vi "CTRE_Phoenix_MotorControl_BufferedTrajectoryPointStream_WriteCCI.vi"(8 "error in":errorcluster, 10 "Trajectory Point":T2, 11 "BufferedTrajectoryPointStream_DevRef":T1) -> (0 "error out":errorcluster, 3 "BufferedTrajectoryPointStream_DevRef":T1)   [LabVIEW 2020]
uses:
  <vilib>/Rock Robotics/WPI/ThirdParty/Phoenix-LabVIEW/Motor Controller/Controls/CTRE_Phoenix_MotorControl_MotionProfileTrajectoryPoint.ctl
  <vilib>/Rock Robotics/WPI/ThirdParty/Phoenix-LabVIEW/Motor Controller/Controls/CTRE_Phoenix_MotorControl_BufferedTrajectoryPointStream_DeviceRef.ctl
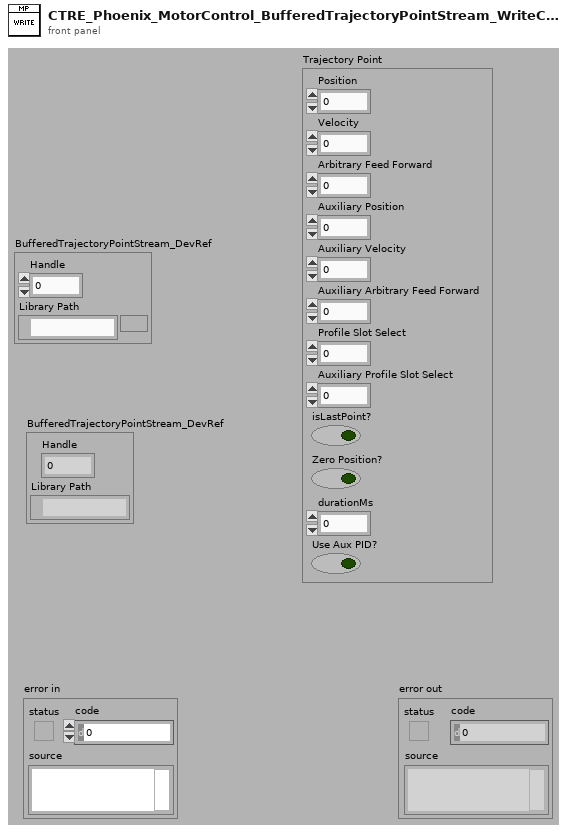
[diagram p1: front panel]
types:
  T1 = typedef "CTRE_Phoenix_MotorControl_BufferedTrajectoryPointStream_DeviceRef.ctl" = cluster{"Handle":u64, "Library Path":path}
  T2 = typedef "CTRE_Phoenix_MotorControl_MotionProfileTrajectoryPoint.ctl" = cluster{"Position":dbl, "Velocity":dbl, "Arbitrary Feed Forward":dbl, "Auxiliary Position":dbl, "Auxiliary Velocity":dbl, "Auxiliary Arbitrary Feed Forward":dbl, "Profile Slot Select":i32, "Auxiliary Profile Slot Select":i32, "isLastPoint?":bool, "Zero Position?":bool, "durationMs":u32, "Use Aux PID?":bool}
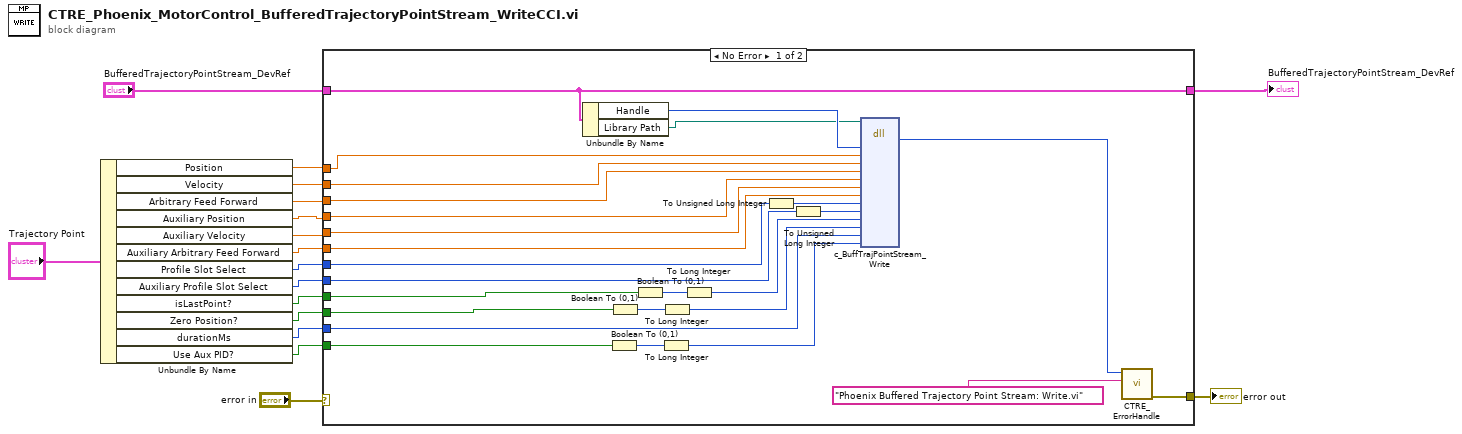
[diagram p0: block diagram]
diagram:
  n1 = Unbundle By Name("Trajectory Point") -> ("Position"=w14:dbl, "Velocity"=w13:dbl, "Arbitrary Feed Forward"=w12:dbl, "Auxiliary Position"=w11:dbl, "Auxiliary Velocity"=w10:dbl, "Auxiliary Arbitrary Feed Forward"=w9:dbl, "Profile Slot Select"=w8:i32, "Auxiliary Profile Slot Select"=w7:i32, "isLastPoint?"=w6:bool, "Zero Position?"=w5:bool, "durationMs"=w4:u32, "Use Aux PID?"=w3:bool)
  n2 = case shown="No Error" "error in" {
    selector: "error in" -> [_ w44]
    tunnel: "BufferedTrajectoryPointStream_DevRef" -> [w20 w45]
    tunnel: [w43 w44] -> w17
    tunnel: [w20 w45] -> w1
    tunnel: w8 -> [w30 _]
    tunnel: w6 -> [w40 _]
    tunnel: w5 -> [w38 _]
    tunnel: w14 -> [w36 _]
    tunnel: w13 -> [w35 _]
    tunnel: w11 -> [w34 _]
    tunnel: w7 -> [w29 _]
    tunnel: w4 -> [w24 _]
    tunnel: w12 -> [w33 _]
    tunnel: w10 -> [w32 _]
    tunnel: w9 -> [w31 _]
    tunnel: w3 -> [w22 _]
    frame No Error {
      n3 = Unbundle By Name(w20) -> ("Handle"=w19:u64, "Library Path"=w18:path)
      n4 = Boolean To (0,1)(Boolean=w22) -> (0, 1=w23:i16)
      n5 = Boolean To (0,1)(Boolean=w38) -> (0, 1=w37:i16)
      n6 = Boolean To (0,1)(Boolean=w40) -> (0, 1=w39:i16)
      n7 = To Long Integer(number=w23) -> (32bit integer=w21:i32)
      n8 = To Long Integer(number=w37) -> (32bit integer=w25:i32)
      n9 = To Long Integer(number=w39) -> (32bit integer=w26:i32)
      n10 = To Unsigned Long Integer(number=w30) -> (unsigned 32bit integer=w28:u32)
      n11 = To Unsigned Long Integer(number=w29) -> (unsigned 32bit integer=w27:u32)
      n12 = dll-call lib="?" fn="c_BuffTrajPointStream_Write"(path in=w18, "handle"=w19, "position"=w36, "velocity"=w35, "arbFeedFwd"=w33, "auxiliaryPos"=w34, "auxiliaryVel"=w32, "auxiliaryArbFeedFwd"=w31, "profileSlotSelect0"=w28, "profileSlotSelect1"=w27, "isLastPoint"=w26, "zeroPos"=w25, "durationMs"=w24, "useAuxPID"=w21) -> ("ErrorCode"=w42:i32)  [unwired: 15 in, 2 out]
      n13 = call <vilib>:"CTRE_ErrorHandle.vi"("origin"="Phoenix Buffered Trajectory Point Stream: Write.vi", "code"=w42) -> ("error out"=w43:errorcluster)  [unwired: 9 in]
    }
    frame Error {
    }
  }
  "error out" <- w17
  "BufferedTrajectoryPointStream_DevRef" <- w1
